vi "RescaleAxis.vi"(0 "pixels in x":i16=250, 1 "pixels in y":i16=200, 5 "Axis scaling Params":T1 {"Y high" format="%.2f"; "Y low" format="%.2f"; "X left" format="%.2f"; "X right" format="%.2f"}, 12 "x":dbl[][](array[numeric]) format="%.2f", 13 "y":dbl[][](array[numeric]) format="%.2f") -> (4 "x scaled":dbl[][](array[numeric]) format="%.2f", 6 "y scaled":dbl[][](array[numeric]) format="%.2f")   [LabVIEW 2022 SP3]
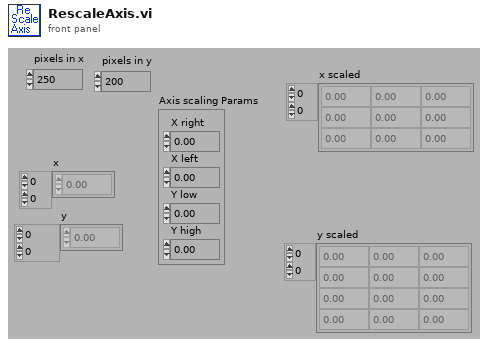
[diagram p1: front panel]
types:
  T1 = cluster{"X right":dbl, "X left":dbl, "Y low":dbl, "Y high":dbl}
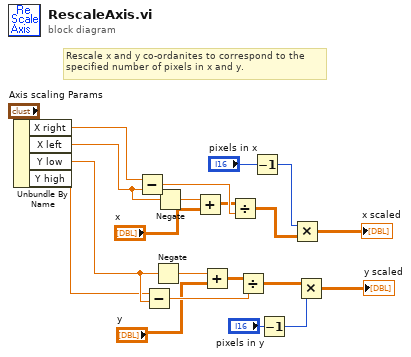
[diagram p0: block diagram]
diagram:
  # "Rescale x and y co-ordanites to correspond to the\nspecified number of pixels in x and y."
  n1 = Unbundle By Name("Axis scaling Params") -> ("X right"=w11:dbl, "X left"=w10:dbl, "Y low"=w9:dbl, "Y high"=w8:dbl)
  n2 = Subtract(x=w11, y=w10) -> (x-y=w21:dbl)
  n3 = Subtract(x=w8, y=w9) -> (x-y=w20:dbl)
  n4 = Negate(x=w9) -> (-x=w14:dbl)
  n5 = Negate(x=w10) -> (-x=w16:dbl)
  n6 = Add(x=w16, y="x") -> (x+y=w17:dbl[][])
  n7 = Add(x=w14, y="y") -> (x+y=w15:dbl[][])
  n8 = Divide(x=w17, y=w21) -> (x/y=w19:dbl[][])
  n9 = Divide(x=w15, y=w20) -> (x/y=w18:dbl[][])
  n10 = Decrement(x="pixels in x") -> (x-1=w2:i16)
  n11 = Decrement(x="pixels in y") -> (x-1=w1:i16)
  n12 = Multiply(x=w2, y=w19) -> (x*y=→"x scaled":dbl[][])
  n13 = Multiply(x=w18, y=w1) -> (x*y=→"y scaled":dbl[][])
